vi "Generate Log String.vi"(7 "Log":string, 8 "error in (no error)":errorcluster, 11 "Process Name":string) -> (0 "error out":errorcluster, 3 "Log String":string)   [LabVIEW 2015, in "Circular Error Log.lvclass"]
uses:
  Circular Error Log.lvclass
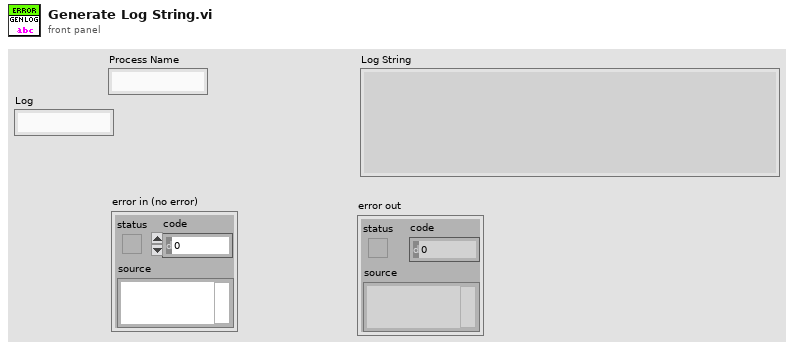
[diagram p1: front panel]
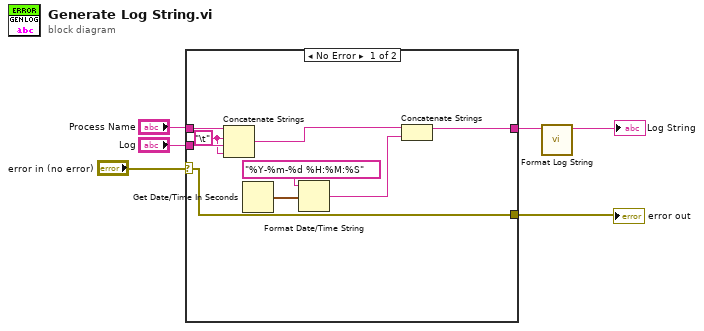
[diagram p0: block diagram]
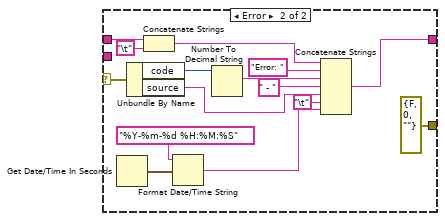
[diagram p2: hidden frame]
diagram:
  n1 = case shown="No Error" "error in (no error)" {
    selector: "error in (no error)" -> [w15 w29]
    tunnel: [w15 errorcluster {"status"=FALSE, "code"=0, "source"=""} ("error IO")] -> w6
    tunnel: "Process Name" -> [w11 w23]
    tunnel: [w14 w16] -> w2
    tunnel: "Log" -> [w10 _]
    frame No Error {
      w9 = "\t"
      n2 = Concatenate Strings(w11, w9, w10, w9) -> (w8:string)
      n3 = Get Date/Time In Seconds() -> (seconds since 1Jan1904=w13:timestamp)
      n4 = Format Date/Time String(time format string (%c)="%Y-%m-%d %H:%M:%S", seconds (now)=w13) -> (date/time string=w7:string)  [unwired: 1 in]
      n5 = Concatenate Strings(w8, w7) -> (w14:string)
    }
    frame Error {
      n6 = Get Date/Time In Seconds() -> (seconds since 1Jan1904=w19:timestamp)
      n7 = Unbundle By Name(w29) -> ("code"=w30:i32, "source"=w25:string)
      n8 = Concatenate Strings(w23, "\t") -> (w21:string)
      n9 = Format Date/Time String(time format string (%c)="%Y-%m-%d %H:%M:%S", seconds (now)=w19) -> (date/time string=w17:string)  [unwired: 1 in]
      n10 = Number To Decimal String(number=w30) -> (decimal integer string=w28:string)  [unwired: 1 in]
      n11 = Concatenate Strings(w21, "Error: " ("string"), w28, " - " ("string"), w25, "\t", w17) -> (w16:string)
    }
  }
  "error out" <- w6
  n12 = call "Format Log String.vi"("Log String In"=w2) -> ("Log String"=→"Log String":string)  [unwired: 10 in]
